vi "Draw Robot XY Graph.vi"(11 "Pose":cluster{"x":dbl, "y":dbl, "theta":dbl}) -> (3 "Robot Pose":cluster{cluster{dbl, dbl}[]}[](graph))   [LabVIEW 2023]
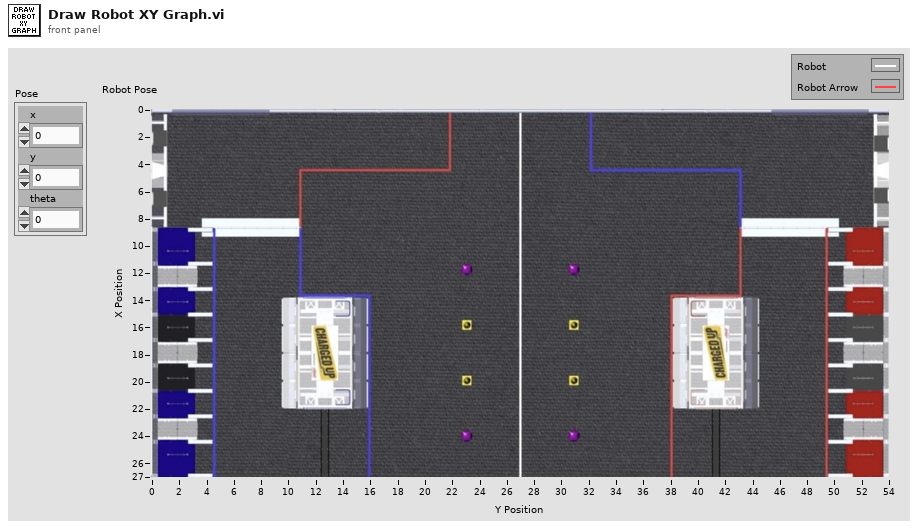
[diagram p1: front panel]
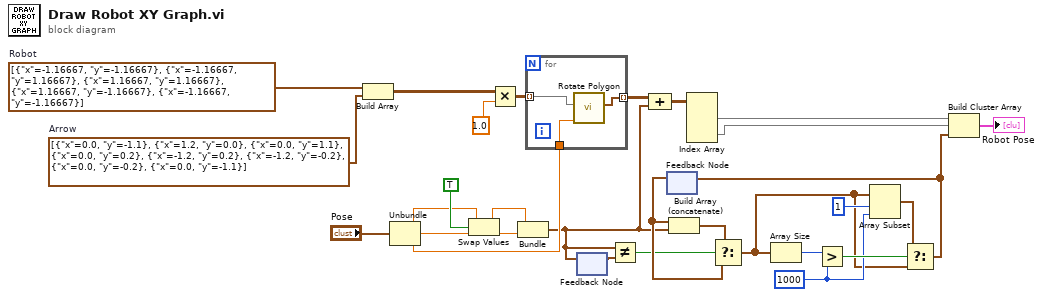
[diagram p0: block diagram]
diagram:
  w10 = 1000 ("y")
  w27 = cluster{"x":dbl, "y":dbl}[] [{"x"=-1.16667, "y"=-1.16667}, {"x"=-1.16667, "y"=1.16667}, {"x"=1.16667, "y"=1.16667}, {"x"=1.16667, "y"=-1.16667}, {"x"=-1.16667, "y"=-1.16667}]  # Robot
  w26 = cluster{"x":dbl, "y":dbl}[] [{"x"=0.0, "y"=-1.1}, {"x"=1.2, "y"=0.0}, {"x"=0.0, "y"=1.1}, {"x"=0.0, "y"=0.2}, {"x"=-1.2, "y"=0.2}, {"x"=-1.2, "y"=-0.2}, {"x"=0.0, "y"=-0.2}, {"x"=0.0, "y"=-1.1}]  # Arrow
  n1 = Build Array(w27, w26) -> (w25:cluster{"x":dbl, "y":dbl}[][])
  n2 = Unbundle("Pose") -> ("x"=w14:dbl, "y"=w19:dbl, "theta"=w15:dbl)
  n3 = Swap Values(12:w14, 13:TRUE ("?(T)"), 14:w19) -> (1:w17:dbl, 3:w16:dbl)
  n4 = Multiply(x=w25, y=1.0 ("Scale")) -> (x*y=w28:cluster{"x":dbl, "y":dbl}[][])
  n5 = Bundle(w17, w16) -> (w3:cluster{dbl, dbl})  [unwired: 1 in]
  n6 = for {
    tunnel: w15 -> [w32]
    tunnel: w28 -> [w30] mode=indexing
    tunnel: [w31] -> w1 mode=indexing
    n7 = call "Rotate Polygon.vi"("Angle"=w32, "polygon 2"=w30) -> ("polygon"=w31:cluster{dbl, dbl}[])  [unwired: 9 in]
  }
  n8 = feedback-in #1(w3) -> ()
  n9 = feedback #1() -> (w4:cluster{dbl, dbl})  [unwired: 1 in]
  n10 = Not Equal?(x=w3, y=w4) -> (x != y?=w2:bool)
  n11 = Compound Arithmetic op=ADD(w1, w3) -> (w24:cluster{dbl, dbl}[][])
  n12 = feedback #2() -> (w6:cluster{dbl, dbl}[])  [unwired: 1 in]
  n13 = Build Array (concatenate)(w6, w3) -> (w7:cluster{dbl, dbl}[])
  n14 = Index Array(array=w24) -> (element #1=w22:cluster{dbl, dbl}[], element #2=w21:cluster{dbl, dbl}[])  [unwired: 4 in]
  n15 = Select(t=w7, s=w2, f=w6) -> (s? t:f=w5:cluster{dbl, dbl}[])
  n16 = Array Size(array=w5) -> (size(s)=w13:i32)
  n17 = Greater?(x=w13, y=w10) -> (0:w12:bool)
  n18 = Array Subset(array=w5, index=1, length=w10) -> (w11:cluster{dbl, dbl}[])
  n19 = Select(t=w11, s=w12, f=w5) -> (s? t:f=w8:cluster{dbl, dbl}[])
  n20 = feedback-in #2(w8) -> ()
  n21 = Build Cluster Array(w22, w21, w8) -> (→"Robot Pose":cluster{cluster{dbl, dbl}[]}[])
